vi "Deckblatt_Filename.vi"(8 "Deckblatt Filename":string, 9 "Deckblatt Prefix":string, 10 "PDF Einzelseiten & Start":bool, 11 "Save PDF File Path (Eingang)":path) -> (2 "PDF Einzelseiten & Start out":bool, 3 "Save PDF File Path (Ausgang)":path)   [LabVIEW 2020, in "Linearisierung v2.lvlib" / "Protokoll.lvlib"]
uses:
  Protokoll.lvlib
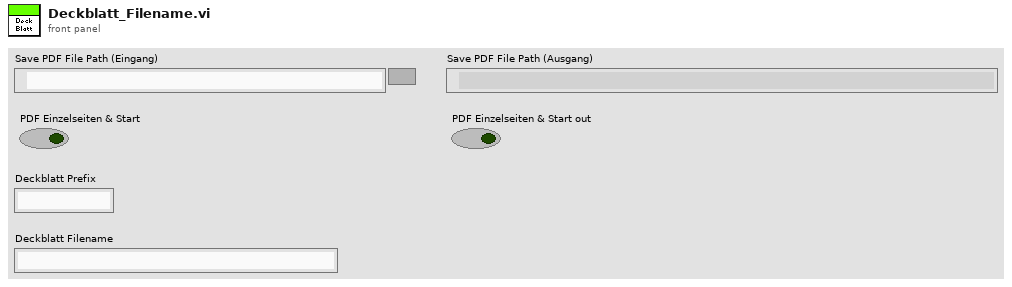
[diagram p1: front panel]
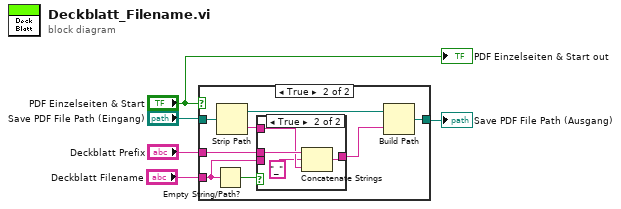
[diagram p0: block diagram]
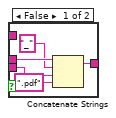
[diagram p3: hidden frame]
diagram:
  n1 = case shown="True" "PDF Einzelseiten & Start" {
    tunnel: "Save PDF File Path (Eingang)" -> [w6 w14]
    tunnel: [w6 w12] -> w5
    tunnel: "Deckblatt Prefix" -> [_ w10]
    tunnel: "Deckblatt Filename" -> [_ w9]
    frame False {
    }
    frame True {
      n2 = Empty String/Path?(string/path=w9) -> (empty?=w11:bool)
      n3 = Strip Path(path=w14) -> (stripped path=w13:path, name=w7:string)
      n4 = case shown="True" w11 {
        tunnel: w10 -> [w18 w23]
        tunnel: w9 -> [w19 _]
        tunnel: [w17 w21] -> w8
        tunnel: w7 -> [_ w22]
        frame False {
          n5 = Concatenate Strings(w18, "_" ("String"), w19, ".pdf" ("String")) -> (w17:string)
        }
        frame True {
          n6 = Concatenate Strings(w23, "_", w22) -> (w21:string)
        }
      }
      n7 = Build Path(base path=w13, name or relative path=w8) -> (appended path=w12:path)
    }
  }
  "Save PDF File Path (Ausgang)" <- w5
  "PDF Einzelseiten & Start out" <- "PDF Einzelseiten & Start"
